vi "HumanSwerveDrive.vi"(9 "Rotation":dbl, 10 "Y":dbl, 11 "X":dbl) -> (1 "A":dbl, 2 "Y":dbl, 3 "X":dbl)   [LabVIEW 2023]
uses:
  <vilib>/Rock Robotics/WPI/ThirdParty/JAS_Junk/TrajLib/Conv_Deg_Radians.vi
  <vilib>/Rock Robotics/WPI/ThirdParty/JAS_Junk/TrajLib/Rotation2d_CreateAngle.vi
  <vilib>/Rock Robotics/WPI/ThirdParty/JAS_Junk/TrajLib/Trajectory_Library.lvlib
panel:
  # "we switched these, hopefully it is right"
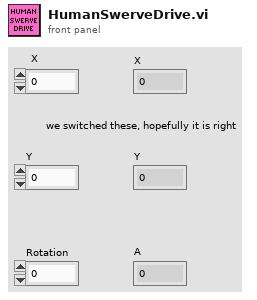
[diagram p1: front panel]
types:
  T1 = typedef "Trajectory_Library.lvlib/ROTATION2D.ctl" = cluster{"VALUE":dbl, "COS":dbl, "SIN":dbl}
  T2 = typedef "Trajectory_Library.lvlib/TRANSLATION2D.ctl" = cluster{"X":dbl, "Y":dbl}
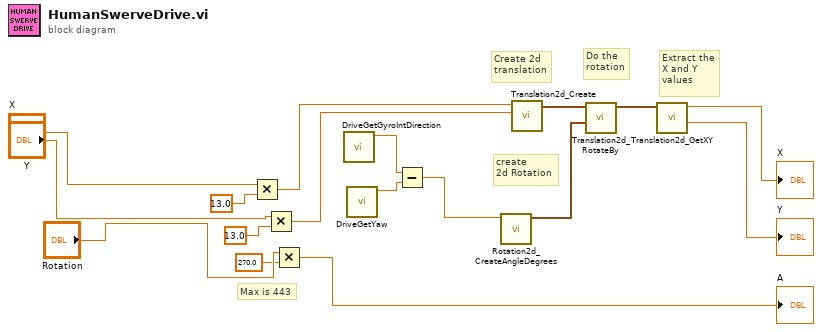
[diagram p0: block diagram]
diagram:
  # "Extract the\nX and Y \nvalues"
  # "Do the \nrotation"
  # "Create 2d\ntranslation"
  # "create\n2d Rotation"
  # "Max is 443"
  n1 = Multiply(x="X", y=13.0) -> (x*y=w10:dbl)
  n2 = Multiply(x="Y", y=13.0) -> (x*y=w11:dbl)
  n3 = Multiply(x="Rotation", y=270.0) -> (x*y=→"A":dbl)
  n4 = call "DriveGetGyroIntDirection.vi"() -> ("GyroIntDirection"=w2:dbl)  [unwired: 11 in]
  n5 = call "DriveGetYaw.vi"() -> ("Yaw"=w1:dbl)  [unwired: 11 in]
  n6 = Subtract(x=w2, y=w1) -> (x-y=w17:dbl)
  n7 = call <vilib>:"Rotation2d_CreateAngleDegrees.vi"("Angle_Degrees"=w17) -> ("ROTATION"=w13:T1)  [unwired: 10 in]
  n8 = call <vilib>:"Translation2d_Create.vi"("Y"=w11, "X"=w10) -> ("TRANSLATION"=w12:T2)  [unwired: 9 in]
  n9 = call <vilib>:"Translation2d_RotateBy.vi"("other Rotation"=w13, "In Translation"=w12) -> ("Out Translation"=w14:T2)  [unwired: 9 in]
  n10 = call <vilib>:"Translation2d_GetXY.vi"("In Translation"=w14) -> ("Y"=→"Y":dbl, "X"=→"X":dbl)  [unwired: 9 in]
